vi "doSTS.vi"(8 "TipLift (m)":sgl format="%#_6p", 9 "milliseconds to wait":u32=1000, 10 "Z Controller setpoint (A)":dbl format="%#_6p", 11 "Bias (V)":sgl=-2.0 format="%_5p") -> ()   [LabVIEW 2014]
uses:
  <userlib>/Nanonis Prog Interface V5/Nanonis Prog Interface.lvlib
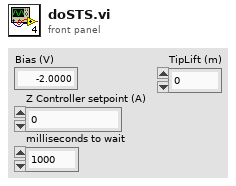
[diagram p1: front panel]
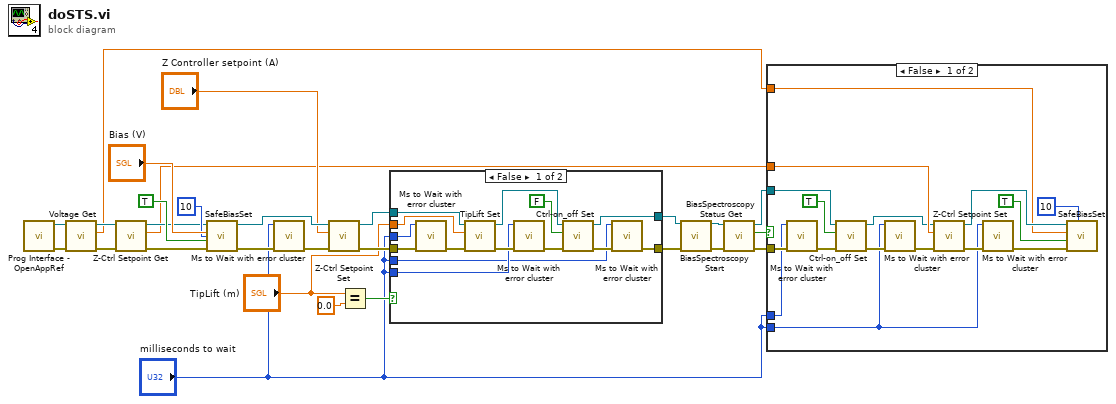
[diagram p0: block diagram]
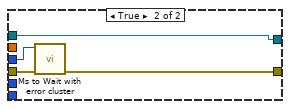
[diagram p2: hidden frame]
diagram:
  n1 = call <userlib>:"Prog Interface - OpenAppRef.vi"() -> ("Error out"=w26:errorcluster, "Application reference"=w27:refnum<vi>)  [unwired: 6 in]
  n2 = call <userlib>:"Voltage Get.vi"("error in (no error)"=w26, "Application ref in"=w27) -> ("error out"=w22:errorcluster, "Bias (V)"=w14:sgl, "Application ref out"=w23:refnum<vi>)  [unwired: 7 in]
  n3 = call <userlib>:"Z-Ctrl Setpoint Get.vi"("error in (no error)"=w22, "Application ref in"=w23) -> ("error out"=w20:errorcluster, "Z Controller setpoint"=w11:sgl, "Application ref out"=w21:refnum<vi>)  [unwired: 6 in]
  n4 = call "SafeBiasSet.vi"("Application ref in"=w21, "Bias (V)"="Bias (V)", "Ramp"=TRUE, "error in (no error)"=w20, "milliseconds to wait"=u32 10) -> ("Application ref out"=w19:refnum<vi>, "Error out"=w10:errorcluster)  [unwired: 4 in]
  n5 = call <userlib>:"Ms to Wait with error cluster.vi"("error in (no error)"=w10, "milliseconds to wait"="milliseconds to wait") -> ("error out"=w9:errorcluster)  [unwired: 4 in, 1 out]
  n6 = call <userlib>:"Z-Ctrl Setpoint Set.vi"("error in (no error)"=w9, "Z Controller setpoint"="Z Controller setpoint (A)", "Application ref in"=w19) -> ("error out"=w5:errorcluster, "Application ref out"=w6:refnum<vi>)  [unwired: 7 in]
  n7 = Equal?(x="TipLift (m)", y=sgl 0.0) -> (x = y?=w7:bool)
  n8 = case shown="False" w7 {
    tunnel: w6 -> [w41 w43]
    tunnel: w5 -> [w39 w46]
    tunnel: [w34 w44] -> w4
    tunnel: [w33 w43] -> w3
    tunnel: "TipLift (m)" -> [w32 _]
    tunnel: "milliseconds to wait" -> [w31 w45]
    tunnel: "milliseconds to wait" -> [w30 _]
    tunnel: "milliseconds to wait" -> [w29 _]
    frame False {
      n9 = call <userlib>:"Ms to Wait with error cluster.vi"("error in (no error)"=w39, "milliseconds to wait"=w31) -> ("error out"=w38:errorcluster)  [unwired: 4 in, 1 out]
      n10 = call <userlib>:"TipLift Set.vi"("error in (no error)"=w38, "TipLift (m)"=w32, "Application ref in"=w41) -> ("error out"=w37:errorcluster, "Application ref out"=w40:refnum<vi>)  [unwired: 7 in]
      n11 = call <userlib>:"Ms to Wait with error cluster.vi"("error in (no error)"=w37, "milliseconds to wait"=w30) -> ("error out"=w36:errorcluster)  [unwired: 4 in, 1 out]
      n12 = call <userlib>:"Ctrl-on_off Set.vi"("error in (no error)"=w36, "Z Controller ON/OFF"=FALSE, "Application ref in"=w40) -> ("error out"=w35:errorcluster, "Application ref out"=w33:refnum<vi>)  [unwired: 7 in]
      n13 = call <userlib>:"Ms to Wait with error cluster.vi"("error in (no error)"=w35, "milliseconds to wait"=w29) -> ("error out"=w34:errorcluster)  [unwired: 4 in, 1 out]
    }
    frame True {
      n14 = call <userlib>:"Ms to Wait with error cluster.vi"("error in (no error)"=w46, "milliseconds to wait"=w45) -> ("error out"=w44:errorcluster)  [unwired: 4 in, 1 out]
    }
  }
  n15 = call <userlib>:"BiasSpectroscopy Start.vi"("Application ref in"=w3, "Error in (no error)"=w4) -> ("Application ref out"=w17:refnum<vi>, "Error out"=w16:errorcluster)  [unwired: 9 in, 3 out]
  n16 = call <userlib>:"BiasSpectroscopy Status Get.vi"("Error in (no error)"=w16, "Application ref in"=w17) -> ("Error out"=w13:errorcluster, "Running?"=w15:bool, "Application ref out"=w12:refnum<vi>)  [unwired: 5 in]
  n17 = case shown="False" w15 {
    tunnel: w14 -> [w58 _]
    tunnel: w13 -> [w57 _]
    tunnel: w12 -> [w52 _]
    tunnel: w11 -> [w60 _]
    tunnel: "milliseconds to wait" -> [w54 _]
    tunnel: "milliseconds to wait" -> [w50 _]
    frame False {
      n18 = call <userlib>:"Ms to Wait with error cluster.vi"("error in (no error)"=w57, "milliseconds to wait"=w54) -> ("error out"=w53:errorcluster)  [unwired: 4 in, 1 out]
      n19 = call <userlib>:"Ctrl-on_off Set.vi"("error in (no error)"=w53, "Z Controller ON/OFF"=TRUE, "Application ref in"=w52) -> ("error out"=w51:errorcluster, "Application ref out"=w48:refnum<vi>)  [unwired: 7 in]
      n20 = call <userlib>:"Ms to Wait with error cluster.vi"("error in (no error)"=w51, "milliseconds to wait"=w50) -> ("error out"=w49:errorcluster)  [unwired: 4 in, 1 out]
      n21 = call <userlib>:"Z-Ctrl Setpoint Set.vi"("error in (no error)"=w49, "Z Controller setpoint"=w60, "Application ref in"=w48) -> ("error out"=w56:errorcluster, "Application ref out"=w59:refnum<vi>)  [unwired: 7 in]
      n22 = call <userlib>:"Ms to Wait with error cluster.vi"("error in (no error)"=w56, "milliseconds to wait"=w50) -> ("error out"=w55:errorcluster)  [unwired: 4 in, 1 out]
      n23 = call "SafeBiasSet.vi"("Application ref in"=w59, "Bias (V)"=w58, "Ramp"=TRUE, "error in (no error)"=w55, "milliseconds to wait"=u32 10) -> ()  [unwired: 4 in, 2 out]
    }
    frame True {
    }
  }
